vi "Write SysCfg Session.vi"(8 "error in":errorcluster, 10 "SysCfg Session":refnum<data-value>, 11 "SysCfg Device in":refnum<class "SysCfg Device.lvclass">) -> (0 "error out":errorcluster, 3 "SysCfg Device out":refnum<class "SysCfg Device.lvclass">)   [LabVIEW 2016, in "SMI.lvlib" / "SysCfg Device.lvclass"]
uses:
  SysCfg Device.lvclass
  SysCfg Device.lvclass/SysCfg Device.ctl
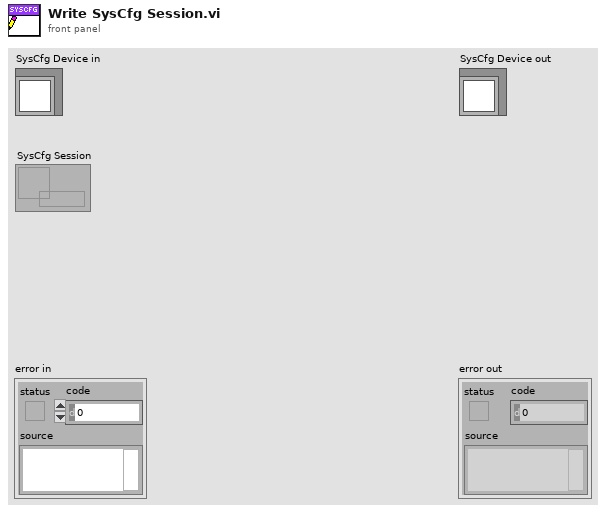
[diagram p1: front panel]
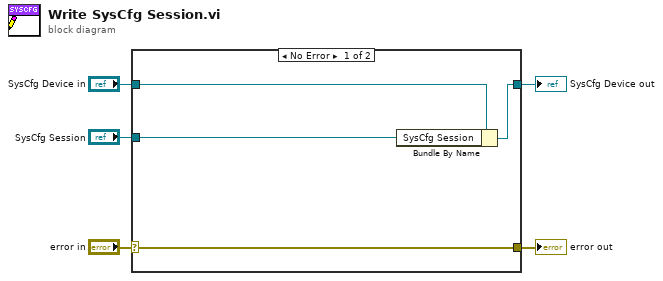
[diagram p0: block diagram]
diagram:
  n1 = case shown="No Error" "error in" {
    selector: "error in" -> [w7 w10]
    tunnel: [w7 w10] -> w4
    tunnel: [w9 w11] -> w2
    tunnel: "SysCfg Device in" -> [w8 w11]
    tunnel: "SysCfg Session" -> [w6 _]
    frame No Error {
      n2 = Bundle By Name(cluster=w8, "SysCfg Session"=w6) -> (w9:refnum<class "SysCfg Device.lvclass">)
    }
    frame Error {
    }
  }
  "error out" <- w4
  "SysCfg Device out" <- w2
